vi "CoordAxis_S.vi"() -> (3 "out Coordinate Axis":T1)   [LabVIEW 2019, in "Trajectory_Library.lvlib"]
doc: "Returns a coordinate axis corresponding to -X in the NWU coordinate system. (South)\n\nInputs: \n -- none --\n\nOutputs:\n - Coordinate Axis -- A data cluster representing a coordinate system axis with respect to the NWU coordinate system."
uses:
  Trajectory_Library.lvlib
  COORDINATE_AXIS.ctl
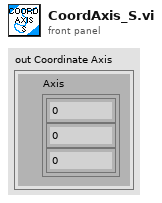
[diagram p1: front panel]
types:
  T1 = typedef "Trajectory_Library.lvlib/COORDINATE_AXIS.ctl" = cluster{"Axis":dbl[]}
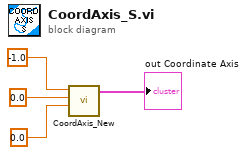
[diagram p0: block diagram]
diagram:
  n1 = call "CoordAxis_New.vi"("Z"=0.0, "Y"=0.0, "X"=-1.0) -> ("out Coordinate Axis"=→"out Coordinate Axis":T1)  [unwired: 8 in]
